vi "LIDAR slave V5.1.vi"() -> ()   [LabVIEW 2015]
uses:
  Controls/AI Slave State.ctl
  Controls/FPGA Nain State.ctl
  <vilib>/Platform/TimedLoop/XDataNode/timing_clust.ctl
  <vilib>/Platform/TimedLoop/XDataNode/nitl_modes.ctl
  <vilib>/Platform/TimedLoop/XDataNode/wakeup.ctl
  <vilib>/rvi/Emulation/niFpgaGetClockAttributes.vi
  <vilib>/rvi/Emulation/niFpgaSctlEmulationGetInTimedLoop.vi
  <vilib>/rvi/Emulation/niFpgaEmulationReportErrorSimple.vi
  LIDAR Slave Globals.vi
  <vilib>/rvi/Emulation/niFpgaProcessEmulError.vi
  <vilib>/rvi/Emulation/niFpgaCriticalErrorInLSC.vi
  <vilib>/rvi/eio/common/nirviEmuTemplateMethod_errors.vi
  <vilib>/rvi/Emulation/niFpgaEmulationIsFPGAContextNoSignature.vi
  <vilib>/rvi/errors/niFpgaSetErrorForExecOnDevCompSimple.vi
  <vilib>/rvi/eio/common/nirviEmuReportErrorAndStop.vi
  <vilib>/rvi/DataTransferAndStorage/Container/Common/niFpgaContainerGetUniqueNameForEmu.vi
  <vilib>/rvi/FIFO/Fifo_Resource/nirvififoEmulationSetSize.vi
  <vilib>/rvi/FIFO/Fifo_Resource/nirviFifoEmulationQueueMgr.vi
  <instcachedir>/0/nirviFifoEmulationQueueMgr_E5CAEC123FF24DC58D834DCA3CDAA9B5.lvgen/nirviFifoEmulationQueueMgr_E5CAEC123FF24DC58D834DCA3CDAA9B5_001.vi
  <vilib>/rvi/FIFO/Fifo_Resource/nirvififoEmulationDetermineInputValidOut.vi
  <vilib>/rvi/FIFO/Fifo_Resource/nirvififoEmulationCreateLock.vi
  <vilib>/rvi/FIFO/Fifo_Resource/nirvififoEmulationObtainLock.vi
  <vilib>/rvi/FIFO/Fifo_Resource/nirvififoEmulationReleaseLock.vi
  <vilib>/rvi/occurrence/nirviWaitOnOccurrenceBase.vi
  <vilib>/rvi/errors/nirviReportUnexpectedCaseInternalError.vi
  <vilib>/rvi/errors/nirviReportUnexpectedCaseInternalError (U32).vi
  <vilib>/Utility/error.llb/Clear Errors.vi
  <vilib>/rvi/interface/RandomDataEmulation/niFpgaRandomDataHandleErrors.vi
  <vilib>/eio/EIONode/EIONode.xnode
  <vilib>/eio/EIOMethodNode/EIOMethodNode.xnode
  <vilib>/Platform/TimedLoop/XDataNode/XDataNode.xnode
  <vilib>/rvi/DataTransferAndStorage/Container/XNode/niFpgaContainer.xnode
  <vilib>/rvi/FIFO/Fifo_Resource/nirvififoEmulationWrite.vi
  <vilib>/rvi/FIFO/Fifo_Resource/nirvififoEmulationRead.vi
  <vilib>/rvi/interface/RandomDataEmulation/nirviRandomDataFpgaReadWriteTemplate.vi
  <vilib>/Platform/TimedLoop/XDataNode/XDNodeRunTimeDep.lvlib
  LIDAR V2 Globals.vi
panel:
  in  "StartSyncAction":bool
  out "Trig1":bool
  in  "SamplesAmount":u16=99
  in  "Debug":bool
  out "SimTrig":bool
  out "PulseIndex":i16=88
  in  "StartAcq":u16=26
  in  "StartES":u16=15
  in  "StopES":u16=30
  out "EnableSignal":bool
  in  "SendAiCMD":u16
  in  "NoOfSamples":u16=99
  in  "EndOfPulseGen":bool=TRUE
  in  "SamplingEnable":bool
  in  "SingleFrame":bool
  out "MainState":T1=enum."ActivatePulseCycle"
  in  "NoOfLeds":u16=95
  in  "PulsePerLed":i16=199
  out "ActiveLedIndex":u16=2
  out "DMATimeout":bool
  in  "ResetTimeout":bool
  in  "DebugValues":bool
  in  "Sample Clock Commit":bool
  in  "Sample Clock Select":u8
  out "SPI Idle":bool
  out "Configuration Error":bool
  out "Synthesizer Locked":bool
  in  "OverrideTrig":bool
  out "VCSL#":u8
  out "SamplesAmpount":u8
  out "FirstIterration":bool
  out "SimSensID":u8
  in  "Mode":bool
  in  "TrigTimeout":u32=10000
  out "AI Slave State":T2=enum."Error"
  # "Simulation"
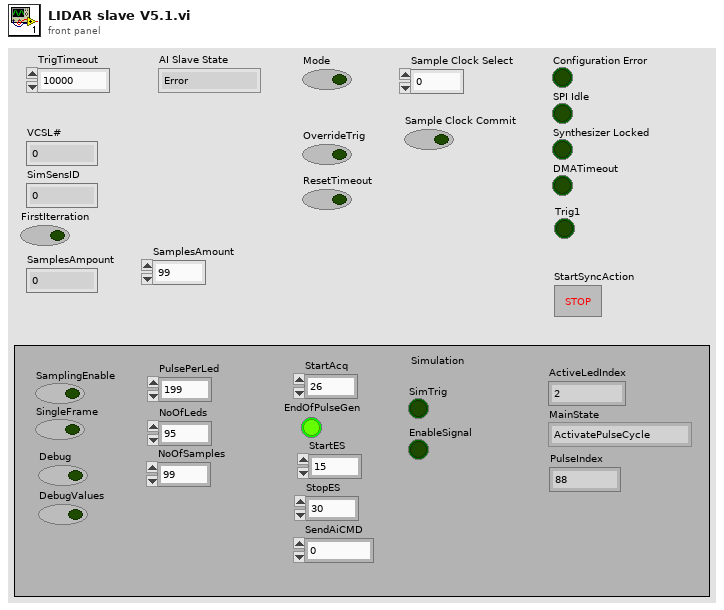
[diagram p1: front panel]
types:
  T1 = typedef "FPGA Nain State.ctl" = enum16{"WaitForStart", "SelectActiveLed", "WaitForNextPulse", "ActivatePulseCycle", "Error"}
  T2 = typedef "AI Slave State.ctl" = enum8{"WaitForStart", "WaitForTrig", "Read AI", "Error"}
  T3 = typedef "XDNodeRunTimeDep.lvlib/timing_clust.ctl" = cluster{"Expected End [f-1]":u64, "Actual End [f-1]":u64, "Finished Late? [f-1]":bool, "Expected End [i-1]":u64, "Actual End [i-1]":u64, "Finished Late? [i-1]":bool, "Expected Start [i]":u64, "Actual Start [i]":u64, "Expected Start [f]":u64, "Actual Start [f]":u64, "Source Name":string, "Structure Name":string, "Period":i64, "Deadline":i64, "Offset":i64, "Start":i64, "Priority":i32, "Timeout":i32, "Mode":T4, "Wakeup Reason":T5, "Error":errorcluster, "Source Type":string, "Secondary Source Type":string, "Global End Time":u64, "Global Start Time":u64, "Frame Duration":u64, "Iteration Duration":u64, "Assigned CPU":i32, "I/O Scan Engine Mode":u32}
  T4 = typedef "XDNodeRunTimeDep.lvlib/nitl_modes.ctl" = enum32{"No Change", "Process missed periods, maintain original phase", "Discard missed periods, maintain original phase", "Process missed periods, ignore original phase", "Discard missed periods, ignore original phase"}
  T5 = typedef "XDNodeRunTimeDep.lvlib/wakeup.ctl" = enum32{"Normal", "Aborted", "Asynchronous wakeup", "Timing source error", "Timed loop error", "Timeout"}
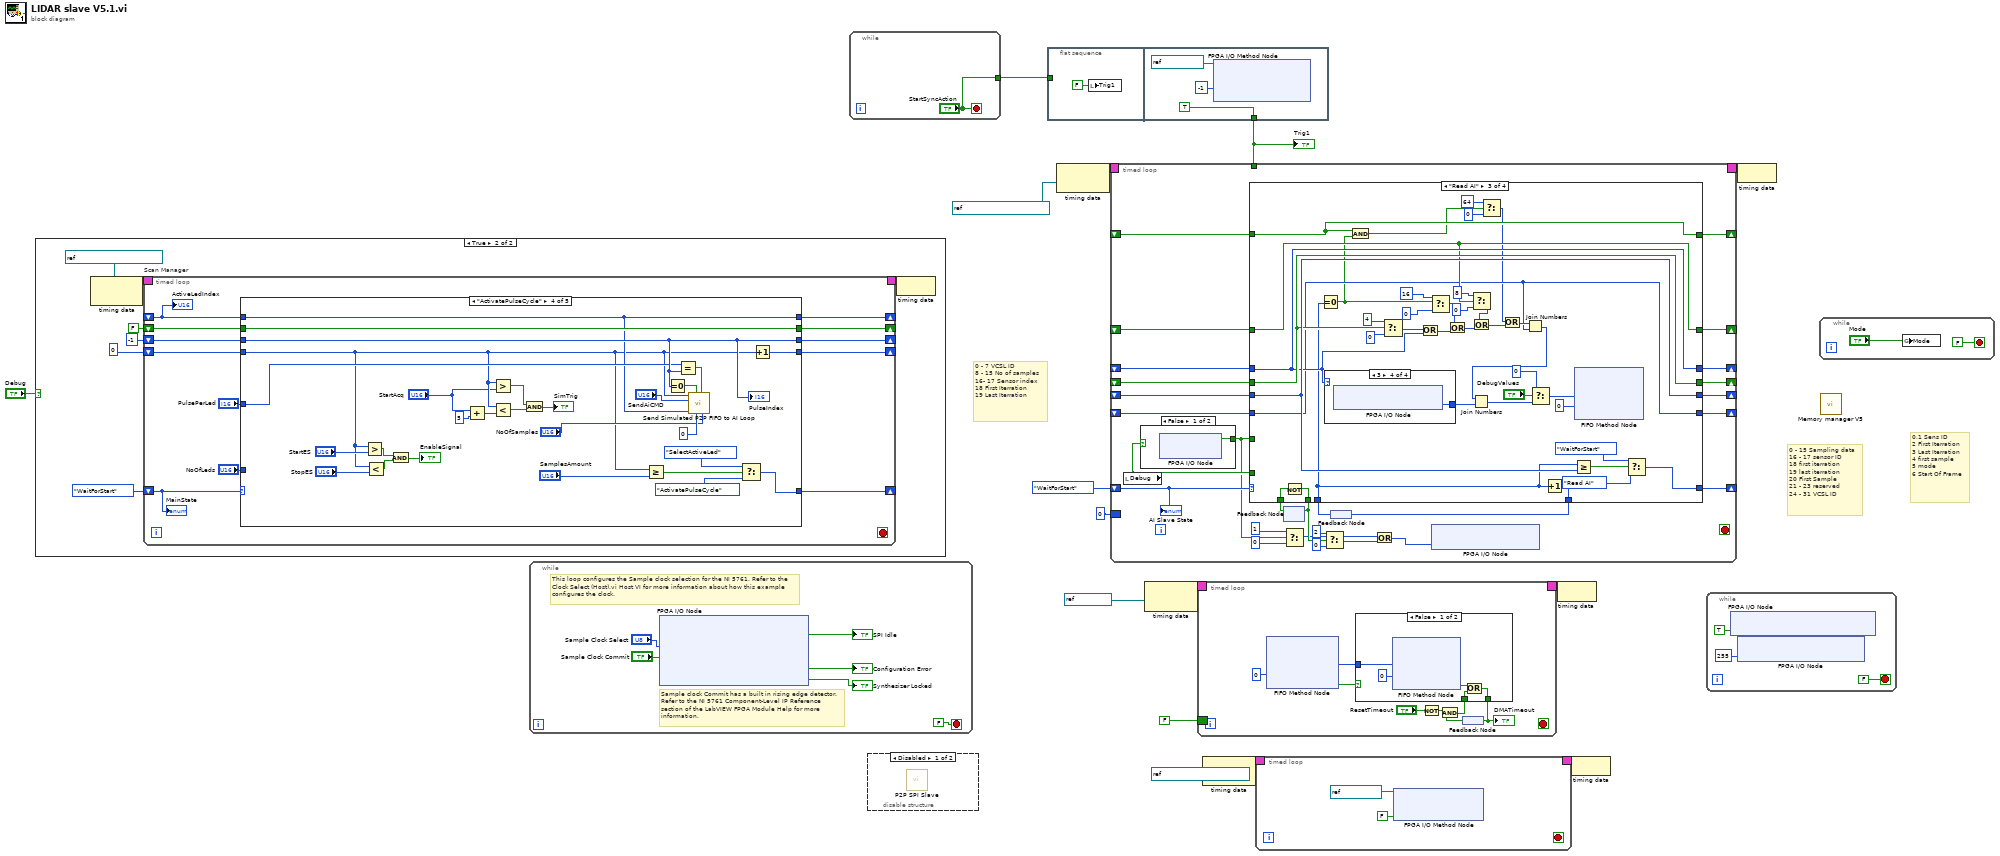
[diagram p0: block diagram]
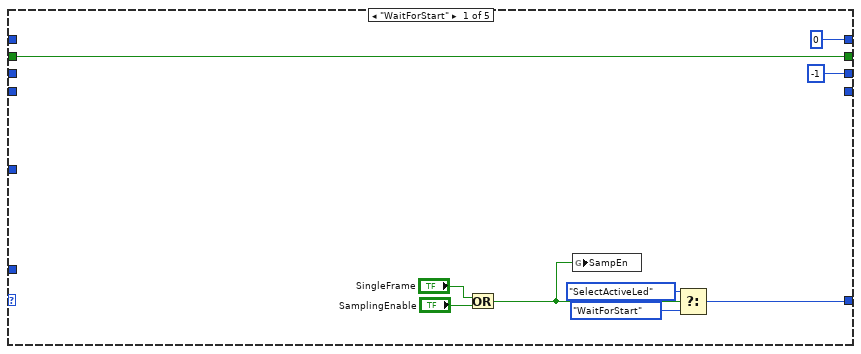
[diagram p4: hidden frame]
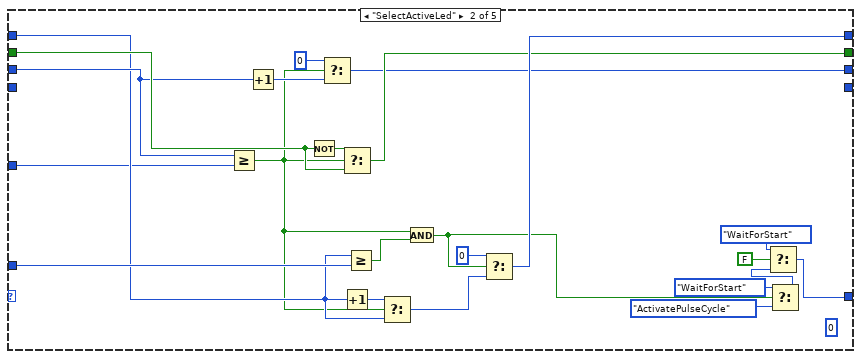
[diagram p5: hidden frame]
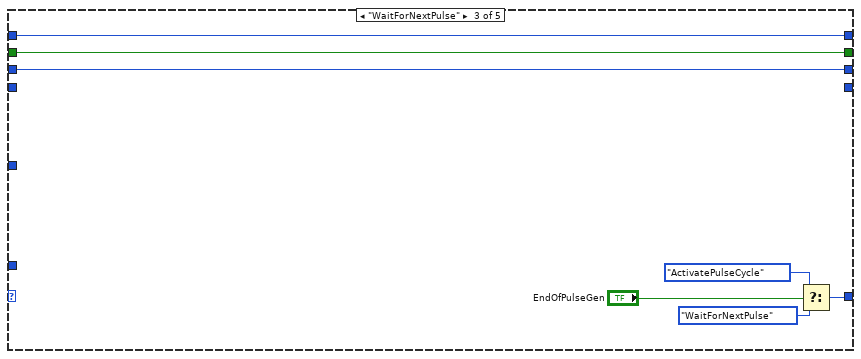
[diagram p6: hidden frame]
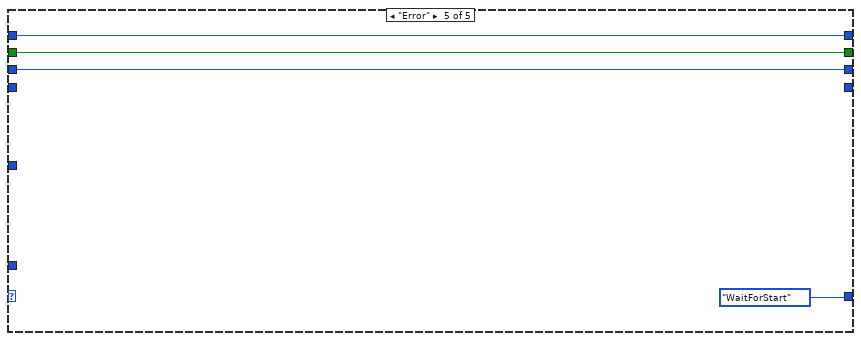
[diagram p7: hidden frame]
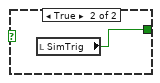
[diagram p9: hidden frame]
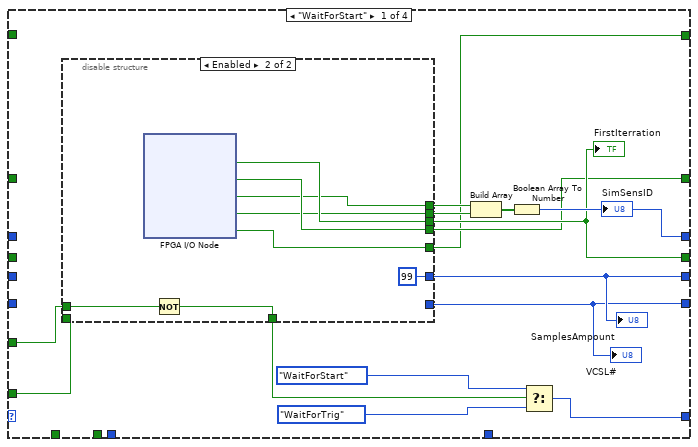
[diagram p10: hidden frame]
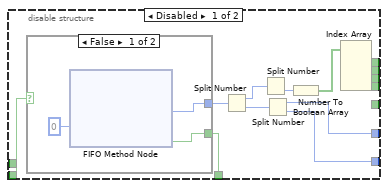
[diagram p11: hidden frame]
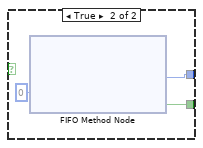
[diagram p12: hidden frame]
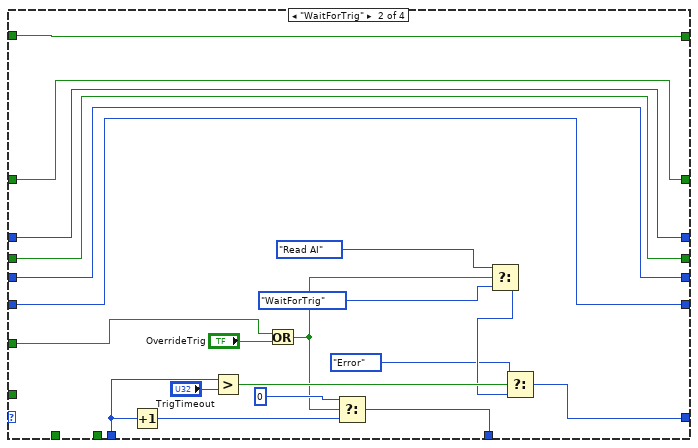
[diagram p13: hidden frame]
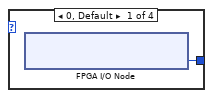
[diagram p14: hidden frame]
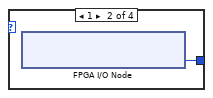
[diagram p15: hidden frame]
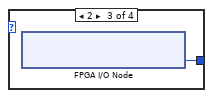
[diagram p16: hidden frame]
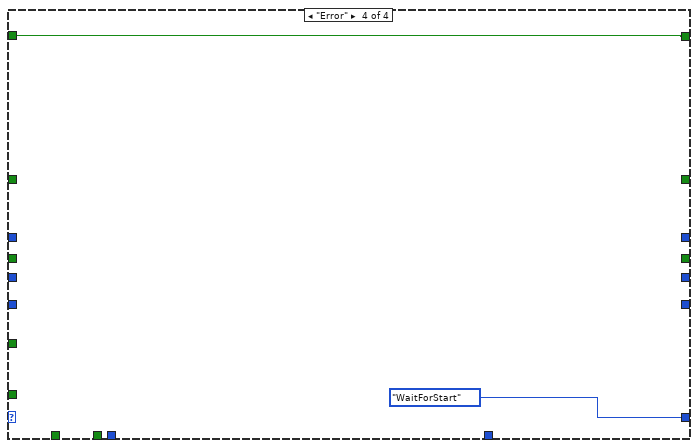
[diagram p17: hidden frame]
diagram:
  # "0,1 Sens ID\n2 First Iterration\n3 Last Iterration\n4 first sample\n5 mode\n6 Start Of Frame"
  # "0 - 15 Sampling data\n16 - 17 sensor ID\n18 first iterration\n19 last iterration\n20 First Sample\n21 - 23 reserved\n24 - 31 VCSL ID"
  # "0 - 7 VCSL ID\n8 - 15 No of samples\n16- 17 Sensor index\n18 First Iterration\n19 Last Iterration"
  n1 = case shown="True" "Debug" {
    frame False {
    }
    frame True {
      n2 = node-c288(refnum<k21> "IO Module\\Data Clock" ("Source Name")) -> (w22:T3)
      n3 = timed-loop "Scan Manager" {
        timing: w22 -> [_]
        timing-out: [_] -> w21
        shift-right: [w33] -> _
        shift-left: FPGA_Nain_State."WaitForStart" ("MainState") -> [w34]
        shift-right: [w28] -> _
        shift-left: _ -> [w23]
        shift-right: [w30] -> _
        shift-left: FALSE -> [w32]
        shift-right: [w31] -> _
        shift-left: i16 -1 -> [w29]
        shift-right: [w24] -> _
        shift-left: u16 0 -> [w25]
        stop <- _ stop-if-true
        n4 = case shown="\"ActivatePulseCycle\"" w34 {
          tunnel: [w41 w63 w69 w97 FPGA_Nain_State."WaitForStart" ("MainState")] -> w33
          tunnel: [u16 0 ("ActiveLedIndex") w59 w68 w84 w104] -> w28
          tunnel: w23 -> [_ w51 w68 w84 w104]
          tunnel: [w38 w58 w73 w96 w103] -> w30
          tunnel: w32 -> [w38 w61 w73 w96 w103]
          tunnel: [i16 -1 ("t") w54 w72 w89 w102] -> w31
          tunnel: w29 -> [_ w57 w72 w89 w102]
          tunnel: "NoOfLeds" -> [_ w53 _ _ _]
          tunnel: "PulsePerLed" -> [_ w44 _ w88 _]
          tunnel: w25 -> [_ _ _ w77 _]
          tunnel: [_ _ _ w95 _] -> w24
          frame "WaitForStart" {
            n5 = Or(x="SingleFrame", y="SamplingEnable") -> (x .or. y?=w35:bool)
            n6 = global write "LIDAR V2 Globals.vi" "SampEn"(w35) -> ()
            n7 = Select(t=FPGA_Nain_State."SelectActiveLed" ("MainState"), s=w35, f=FPGA_Nain_State."WaitForStart" ("MainState")) -> (s? t:f=w41:T1)
          }
          frame "SelectActiveLed" {
            (unwired) u8 0
            n8 = Greater Or Equal?(x=w57, y=w44) -> (x >= y?=w46:bool)
            n9 = Increment(x=w57) -> (x+1=w56:i16)
            n10 = Not(x=w61) -> (.not. x?=w60:bool)
            n11 = Select(t=i16 0, s=w46, f=w56) -> (s? t:f=w54:i16)
            n12 = Select(t=w60, s=w46, f=w61) -> (s? t:f=w58:bool)
            n13 = Increment(x=w51) -> (x+1=w49:u16)
            n14 = Greater Or Equal?(x=w51, y=w53) -> (x >= y?=w47:bool)
            n15 = Select(t=w49, s=w46, f=w51) -> (s? t:f=w50:u16)
            n16 = And(x=w46, y=w47) -> (x .and. y?=w45:bool)
            n17 = Select(t=u16 0, s=w45, f=w50) -> (s? t:f=w59:u16)
            n18 = Select(t=FPGA_Nain_State."WaitForStart" ("MainState"), s=w45, f=FPGA_Nain_State."ActivatePulseCycle" ("MainState")) -> (s? t:f=w64:T1)
            n19 = Select(t=FPGA_Nain_State."WaitForStart" ("MainState"), s=FALSE, f=w64) -> (s? t:f=w63:T1)
          }
          frame "WaitForNextPulse" {
            n20 = Select(t=FPGA_Nain_State."ActivatePulseCycle" ("MainState"), s="EndOfPulseGen", f=FPGA_Nain_State."WaitForNextPulse" ("MainState")) -> (s? t:f=w69:T1)
          }
          frame "ActivatePulseCycle" {
            n21 = Greater?(x=w77, y="StartES") -> (0:w91:bool)
            n22 = Less?(x=w77, y="StopES") -> (x < y?=w92:bool)
            n23 = And(x=w91, y=w92) -> (x .and. y?=→"EnableSignal":bool)
            n24 = Add(x="StartAcq", y=i16 5) -> (x+y=w81:u16)
            n25 = Greater?(x=w77, y="StartAcq") -> (0:w79:bool)
            n26 = Less?(x=w77, y=w81) -> (x < y?=w78:bool)
            n27 = And(x=w79, y=w78) -> (x .and. y?=→"SimTrig":bool)
            n28 = Greater Or Equal?(x=w77, y="SamplesAmount") -> (x >= y?=w100:bool)
            n29 = Equal To 0?(x=w89) -> (x = 0?=w87:bool)
            n30 = Equal?(x=w88, y=w89) -> (x = y?=w86:bool)
            n31 = call "Send Simulated P2P FIFO to AI Loop.vi"("NoOfSamples"="NoOfSamples", "LastIterration"=w86, "SensorID"=u16 0, "FirstIterration"=w87, "ActiveLedIndex"=w84, "SendAiCMD"="SendAiCMD", "TimingCounter"=w77) -> ()  [unwired: 5 in]
            n32 = Select(t=FPGA_Nain_State."SelectActiveLed" ("MainState"), s=w100, f=FPGA_Nain_State."ActivatePulseCycle" ("MainState")) -> (s? t:f=w97:T1)
            n33 = Increment(x=w77) -> (x+1=w95:u16)
            "PulseIndex" <- w89
          }
          frame "Error" {
          }
        }
        "MainState" <- w34
        "ActiveLedIndex" <- w23
      }
      n34 = node-c288(w21) -> ()
    }
  }
  n35 = while {
    stop <- FALSE stop-if-true
    # "Sample clock Commit has a built in rising edge detector. Refer to the NI 5761 Component-Level IP Reference section of the LabVIEW FPGA Module Help for more information."
    # "This loop configures the Sample clock selection for the NI 5761. Refer to the Clock Select (Host).vi Host VI for more information about how this example configures the clock."
    n36 = xnode "FPGA I/O Node"("IO Module\\Sample Clock Select"="Sample Clock Select", "IO Module\\Sample Clock Commit"="Sample Clock Commit") -> ("IO Module\\SPI Idle"=→"SPI Idle":bool, "IO Module\\Configuration Error"=→"Configuration Error":bool, "IO Module\\Synthesizer Locked"=→"Synthesizer Locked":bool)  [unwired: 5 in, 5 out]
  }
  n37 = while {
    tunnel: ["StartSyncAction"] -> w4
    stop <- "StartSyncAction" stop-if-true
  }
  n38 = disable-structure shown="Disabled" {
    frame Disabled {
      n39 = call "P2P SPI Slave.vi"() -> ()  [unwired: 12 in]
    }
    frame Enabled {
    }
  }
  n40 = flat-sequence {
    tunnel: w4 -> [_]
    tunnel: [TRUE] -> w5
    frame #0 {
      n41 = local write "Trig1"(FALSE ("Trig1")) -> ()
    }
    frame #1 {
      n42 = xnode "FPGA I/O Method Node"("FPGA I/O In"=refnum<k21> "PXI_Trig1", "Timeout"=-1) -> ()  [unwired: 2 out]
    }
  }
  n43 = node-c288(refnum<k21> "IO Module\\Data Clock" ("Source Name")) -> (w15:T3)
  n44 = timed-loop {
    timing: w15 -> [_]
    timing-out: [_] -> w14
    shift-right: [w148] -> _
    shift-left: AI_Slave_State."WaitForStart" -> [w137]
    shift-right: [w147] -> _
    shift-left: _ -> [w146]
    shift-right: [w145] -> _
    shift-left: _ -> [w144]
    shift-right: [w143] -> _
    shift-left: _ -> [w142]
    shift-right: [w141] -> _
    shift-left: _ -> [w140]
    border: i16 0 -> [_]
    shift-right: [w136] -> _
    shift-left: _ -> [w135]
    tunnel: w5 -> [_]
    shift-right: [w123] -> _
    shift-left: _ -> [w122]
    stop <- _ stop-if-true
    n45 = local read "Debug"() -> (w134:bool)
    n46 = case shown="False" w134 {
      tunnel: [w149 w150] -> w133
      frame False {
        n47 = xnode "FPGA I/O Node"() -> ("PXI_Trig0"=w149:bool)  [unwired: 1 in, 1 out]
      }
      frame True {
        n48 = local read "SimTrig"() -> (w150:bool)
      }
    }
    n49 = feedback #1() -> (w130:bool)  [unwired: 1 in]
    n50 = Select(t=u8 1, s=w133, f=u8 0) -> (s? t:f=w125:u8)
    n51 = feedback #2() -> (w139:i16)
    n52 = case shown="\"Read AI\"" w137 {
      tunnel: [w162 w201 w245 AI_Slave_State."WaitForStart"] -> w148
      tunnel: [w158 w209 w222 _] -> w147
      tunnel: w146 -> [_ w209 w222 _]
      tunnel: [w159 w210 w249 _] -> w145
      tunnel: w144 -> [_ w210 w249 _]
      tunnel: [w160 w211 w244 _] -> w143
      tunnel: w142 -> [_ w211 w244 _]
      tunnel: [w161 w212 w241 _] -> w141
      tunnel: w140 -> [_ w212 w241 _]
      tunnel: w139 -> [_ w206 w228 _]
      tunnel: [_ w199 w250 _] -> w138
      tunnel: w133 -> [w152 w195 _ _]
      tunnel: [w154 w194 w230 _] -> w136
      tunnel: w135 -> [_ w194 w230 _]
      tunnel: w134 -> [w153 _ _ _]
      tunnel: [_ _ w227 _] -> w127
      tunnel: w130 -> [_ _ w226 _]
      tunnel: [w151 w193 w220 w256] -> w123
      tunnel: w122 -> [_ w193 w220 w256]
      frame "WaitForStart" {
        n53 = disable-structure shown="Enabled" {
          disable-tunnel: [w178 w187] -> w165
          disable-tunnel: [w177 w192] -> w160
          disable-tunnel: [w176 u8 99 ("SamplesAmpount")] -> w159
          disable-tunnel: [w175 _] -> w158
          disable-tunnel: [w169 w190] -> w157
          disable-tunnel: [w168 w189] -> w156
          disable-tunnel: [w167 w191] -> w154
          disable-tunnel: w153 -> [w166 _]
          disable-tunnel: w152 -> [_ w188]
          disable-tunnel: [_ w185] -> w151
          frame Disabled {
            n54 = case shown="False" w166 {
              tunnel: [w180 w182] -> w178
              tunnel: [w181 w183] -> w174
              frame False {
                n55 = xnode ("FIFO Method Node")("Timeout"=0) -> ("Element"=w181:u32, "Timed Out?"=w180:bool)  [unwired: 1 in, 1 out]
              }
              frame True {
                n56 = xnode ("FIFO Method Node")("Timeout"=0) -> ("Element"=w183:u32, "Timed Out?"=w182:bool)  [unwired: 1 in, 1 out]
              }
            }
            n57 = Split Number(x=w174) -> (hi(x)=w172:u16, lo(x)=w173:u16)
            n58 = Split Number(x=w172) -> (lo(x)=w171:u8)  [unwired: 1 out]
            n59 = Split Number(x=w173) -> (hi(x)=w176:u8, lo(x)=w175:u8)
            n60 = Number To Boolean Array(number=w171) -> (Boolean array=w170:bool[])
            n61 = Index Array(array=w170) -> (element #1=w169:bool, element #2=w168:bool, element #3=w177:bool, element #4=w167:bool)  [unwired: 4 in]
          }
          frame Enabled {
            n62 = xnode "FPGA I/O Node"() -> ("PXI_Trig2"=w192:bool, "PXI_Trig3"=w191:bool, "PXI_Trig4"=w190:bool, "PXI_Trig5"=w189:bool, "PXI_Trig6"=w185:bool)  [unwired: 5 in, 5 out]
            n63 = Not(x=w188) -> (.not. x?=w187:bool)
          }
        }
        "FirstIterration" <- w160
        "SamplesAmpount" <- w159
        "VCSL#" <- w158
        n64 = Build Array(w157, w156) -> (w155:bool[])
        n65 = Boolean Array To Number(Boolean array=w155) -> (number=w161:u8)
        "SimSensID" <- w161
        n66 = Select(t=AI_Slave_State."WaitForStart", s=w165, f=AI_Slave_State."WaitForTrig") -> (s? t:f=w162:T2)
      }
      frame "WaitForTrig" {
        n67 = Increment(x=w206) -> (x+1=w200:i16)
        n68 = Greater?(x=w206, y="TrigTimeout") -> (0:w204:bool)
        n69 = Or(x=w195, y="OverrideTrig") -> (x .or. y?=w197:bool)
        n70 = Select(t=i16 0, s=w197, f=w200) -> (s? t:f=w199:i16)
        n71 = Select(t=AI_Slave_State."Read AI", s=w197, f=AI_Slave_State."WaitForTrig") -> (s? t:f=w203:T2)
        n72 = Select(t=AI_Slave_State."Error", s=w204, f=w203) -> (s? t:f=w201:T2)
      }
      frame "Read AI" {
        n73 = Not(x=w226) -> (.not. x?=w227:bool)
        n74 = Equal To 0?(x=w228) -> (x = 0?=w221:bool)
        n75 = case shown="3" w241 {
          tunnel: [w252 w253 w254 w255] -> w216
          frame 0, Default {
            n76 = xnode "FPGA I/O Node"() -> ("IO Module\\AI 0 Data N"=w252:i16)  [unwired: 1 in, 1 out]
          }
          frame 1 {
            n77 = xnode "FPGA I/O Node"() -> ("IO Module\\AI 1 Data N"=w253:i16)  [unwired: 1 in, 1 out]
          }
          frame 2 {
            n78 = xnode "FPGA I/O Node"() -> ("IO Module\\AI 2 Data N"=w254:i16)  [unwired: 1 in, 1 out]
          }
          frame 3 {
            n79 = xnode "FPGA I/O Node"() -> ("IO Module\\AI 3 Data N"=w255:i16)  [unwired: 1 in, 1 out]
          }
        }
        n80 = And(x=w220, y=w221) -> (x .and. y?=w219:bool)
        n81 = Select(t=u8 4, s=w244, f=u8 0) -> (s? t:f=w242:u8)
        n82 = Or(x=w242, y=w241) -> (x .or. y?=w238:u8)
        n83 = Select(t=u8 16, s=w221, f=u8 0) -> (s? t:f=w235:u8)
        n84 = Or(x=w235, y=w238) -> (x .or. y?=w233:u8)
        n85 = Select(t=u8 8, s=w230, f=u8 0) -> (s? t:f=w229:u8)
        n86 = Or(x=w229, y=w233) -> (x .or. y?=w217:u8)
        n87 = Select(t=u8 64, s=w219, f=u8 0) -> (s? t:f=w218:u8)
        n88 = Or(x=w218, y=w217) -> (x .or. y?=w223:u8)
        n89 = Join Numbers(hi=w223, lo=w222) -> ((hi.lo)=w240:u16)
        n90 = Join Numbers(hi=w240, lo=w216) -> ((hi.lo)=w215:u32)
        n91 = Select(t=u32 0, s="DebugValues", f=w215) -> (s? t:f=w214:u32)
        n92 = Increment(x=w228) -> (x+1=w250:i16)
        n93 = Greater Or Equal?(x=w228, y=w249) -> (x >= y?=w248:bool)
        n94 = xnode ("FIFO Method Node")("Element"=w214, "Timeout"=0) -> ()  [unwired: 1 in, 2 out]
        n95 = Select(t=AI_Slave_State."WaitForStart", s=w248, f=AI_Slave_State."Read AI") -> (s? t:f=w245:T2)
      }
      frame "Error" {
      }
    }
    n96 = feedback-in #1(w127) -> ()
    n97 = Select(t=u8 2, s=w127, f=u8 0) -> (s? t:f=w126:u8)
    n98 = feedback-in #2(w138) -> ()
    n99 = Or(x=w125, y=w126) -> (x .or. y?=w124:u8)
    n100 = xnode "FPGA I/O Node"("IO Module\\PFI Output"=w124) -> ()  [unwired: 1 in, 1 out]
    "AI Slave State" <- w137
  }
  n101 = node-c288(refnum<k21> "130MHz" ("Source Name")) -> (w10:T3)
  n102 = timed-loop {
    timing: w10 -> [_]
    timing-out: [_] -> w9
    border: FALSE -> [_]
    stop <- _ stop-if-true
    n103 = xnode ("FIFO Method Node")("Timeout"=0) -> ("Element"=w265:u32, "Timed Out?"=w267:bool)  [unwired: 1 in, 1 out]
    n104 = Not(x="ResetTimeout") -> (.not. x?=w260:bool)
    n105 = feedback #3() -> (w262:bool)
    n106 = And(x=w260, y=w262) -> (x .and. y?=w263:bool)
    n107 = case shown="False" w267 {
      tunnel: w265 -> [w272 _]
      tunnel: [w269 w273] -> w264
      tunnel: w263 -> [w268 w273]
      frame False {
        n108 = xnode ("FIFO Method Node")("Element"=w272, "Timeout"=0) -> ("Timed Out?"=w270:bool)  [unwired: 1 in, 1 out]
        n109 = Or(x=w270, y=w268) -> (x .or. y?=w269:bool)
      }
      frame True {
      }
    }
    "DMATimeout" <- w264
    n110 = feedback-in #3(w264) -> ()
  }
  n111 = node-c288(refnum<k21> "IO Module\\Data Clock" ("Source Name")) -> (w3:T3)
  n112 = timed-loop {
    timing: w3 -> [_]
    timing-out: [_] -> w2
    stop <- _ stop-if-true
    n113 = xnode "FPGA I/O Method Node"("FPGA I/O In"=refnum<k21> "PXI_Trig0", "Enable"=FALSE) -> ()  [unwired: 1 out]
  }
  n114 = node-c288(w9) -> ()
  n115 = node-c288(w2) -> ()
  n116 = while {
    stop <- FALSE stop-if-true
    n117 = xnode "FPGA I/O Node"("IO Module\\PFI Connector Enable"=TRUE ("IO Module\\PFI Connector Enable")) -> ()  [unwired: 1 in, 1 out]
    n118 = xnode "FPGA I/O Node"("IO Module\\PFI Write Enable"=u8 255 ("IO Module\\PFI Write Enable")) -> ()  [unwired: 1 in, 1 out]
  }
  n119 = node-c288(w14) -> ()
  n120 = while {
    stop <- FALSE stop-if-true
    n121 = global write "LIDAR Slave Globals.vi" "Mode"("Mode") -> ()
  }
  n122 = call "Memory manager V5.vi"() -> ()  [unwired: 12 in]
  "Trig1" <- w5
